vi "highest motor value lexi.vi"(1 "motor value":dbl(slide) scale=-619.0..1000.0) -> (0 "...highest value":dbl)   [LabVIEW 2019]
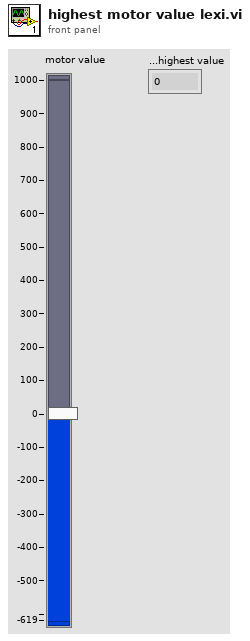
[diagram p1: front panel]
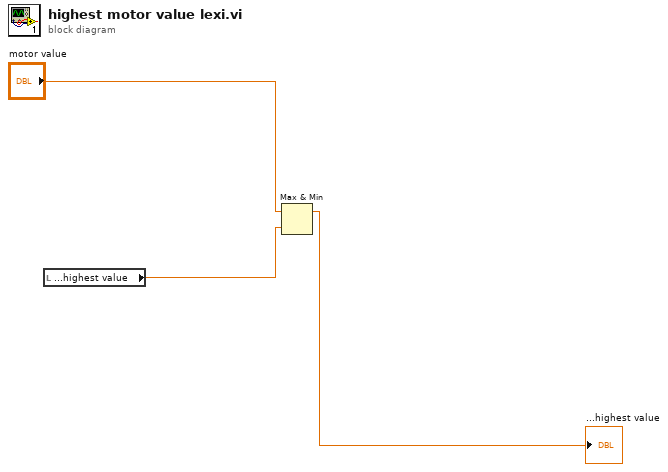
[diagram p0: block diagram]
diagram:
  n1 = local read "...highest value"() -> (w1:dbl)
  n2 = Max & Min(x="motor value", y=w1) -> (max(x,y)=→"...highest value":dbl)  [unwired: 1 out]
